vi "CAN Jaguar Get Status.vi"(8 "error in (no error)":errorcluster, 10 "Status Select":T1[](array[typedef])=[enum."Voltage"], 11 "CAN Jaguar Ref":T3={"Device Number"=0, "Control Mode"=enum."Percent VBus", "Inverted"=FALSE, "Semaphore"=refnum, "Max Vout"=12.0, "DevStatus"={"status"=FALSE, "code"=0, "source"=""}}) -> (0 "error out":errorcluster, 2 "Status":T2, 3 "CAN Jaguar Ref Out":T3={"Device Number"=0, "Control Mode"=enum."Percent VBus", "Inverted"=FALSE, "Semaphore"=refnum, "Max Vout"=12.0, "DevStatus"={"status"=FALSE, "code"=0, "source"=""}})   [LabVIEW 2009, in "CAN.lvlib"]
uses:
  CAN.lvlib
  SubVIs/CAN Jaguar Ref.ctl
  SubVIs/CAN Jaguar Control Mode.ctl
  SubVIs/CAN Jaguar Status.ctl
  SubVIs/CAN Jaguar Status Select.ctl
  SubVIs/CAN Motor Message IDs.ctl
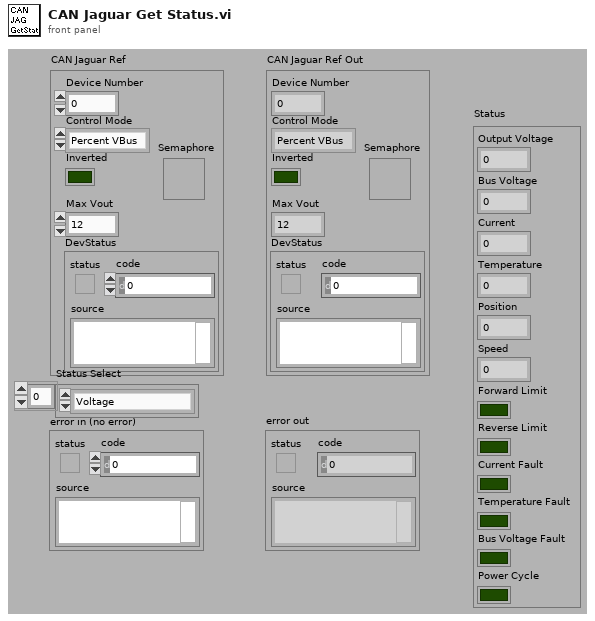
[diagram p1: front panel]
types:
  T1 = typedef "CAN.lvlib/CAN Jaguar Status Select.ctl" = enum16{"Voltage", "Current", "Temperature", "Position", "Speed", "Limit Switches", "Faults", "Power Cycle"}
  T2 = typedef "CAN.lvlib/CAN Jaguar Status.ctl" = cluster{"Output Voltage":dbl, "Bus Voltage":dbl, "Current":dbl, "Temperature":dbl, "Position":dbl, "Speed":dbl, "Forward Limit":bool, "Reverse Limit":bool, "Current Fault":bool, "Temperature Fault":bool, "Bus Voltage Fault":bool, "Power Cycle":bool}
  T3 = typedef "CAN.lvlib/CAN Jaguar Ref.ctl" = cluster{"Device Number":u8, "Control Mode":T4, "Inverted":bool, "Semaphore":T5, "Max Vout":dbl, "DevStatus":errorcluster}
  T4 = typedef "CAN.lvlib/CAN Jaguar Control Mode.ctl" = enum16{"Percent VBus", "Speed", "Position", "Current"}
  T5 = typedef "Semaphore RefNum" = refnum<k1>
  T6 = enum16{"big-endian, network order", "native, host order", "little-endian"}
  T7 = typedef "CAN Jaguar Status.ctl" = cluster{"Output Voltage":dbl, "Bus Voltage":dbl, "Current":dbl, "Temperature":dbl, "Position":dbl, "Speed":dbl, "Forward Limit":bool, "Reverse Limit":bool, "Current Fault":bool, "Temperature Fault":bool, "Bus Voltage Fault":bool, "Power Cycle":bool}
  T8 = typedef "CAN.lvlib/CAN Motor Message IDs.ctl" = u32
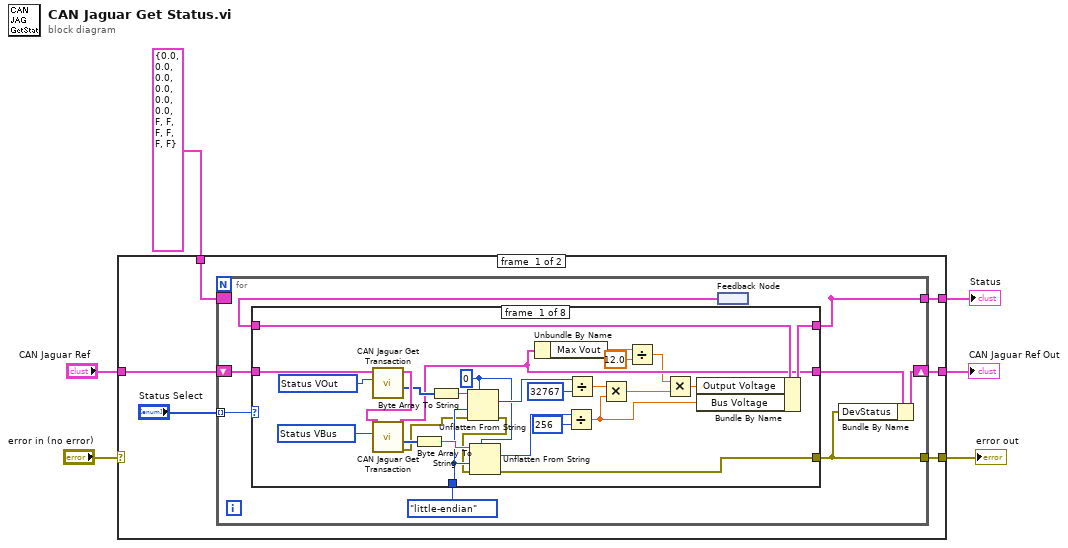
[diagram p0: block diagram]
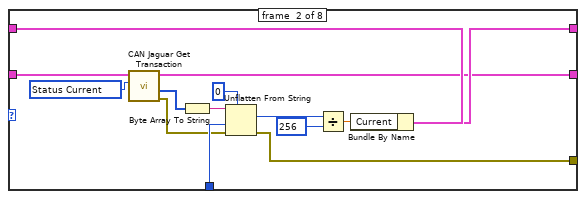
[diagram p2: hidden frame]
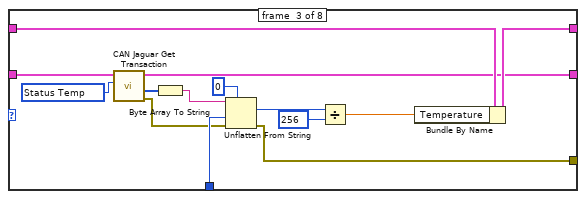
[diagram p3: hidden frame]
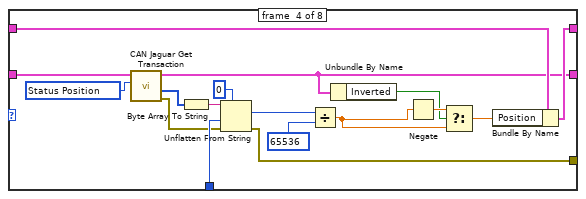
[diagram p4: hidden frame]
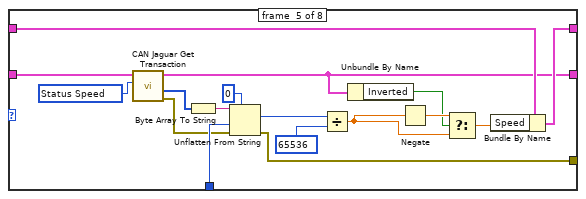
[diagram p5: hidden frame]
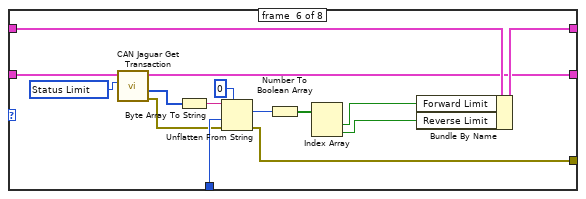
[diagram p6: hidden frame]
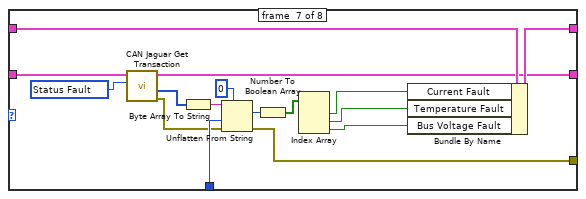
[diagram p7: hidden frame]
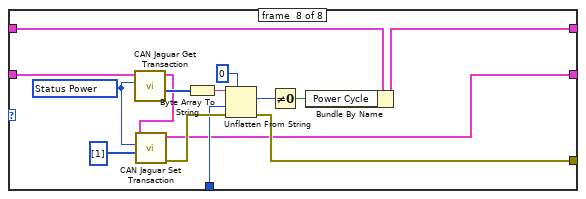
[diagram p8: hidden frame]
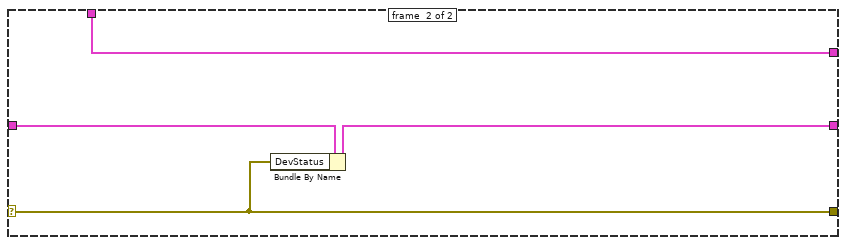
[diagram p9: hidden frame]
diagram:
  n1 = case shown="No Error" "error in (no error)" {
    selector: "error in (no error)" -> [_ w157]
    tunnel: [w7 w158] -> w6
    tunnel: "CAN Jaguar Ref" -> [w8 w159]
    tunnel: [w12 w157] -> w4
    tunnel: T2 {"Output Voltage"=0.0, "Bus Voltage"=0.0, "Current"=0.0, "Temperature"=0.0, "Position"=0.0, "Speed"=0.0, "Forward Limit"=FALSE, "Reverse Limit"=FALSE, "Current Fault"=FALSE, "Temperature Fault"=FALSE, "Bus Voltage Fault"=FALSE, "Power Cycle"=FALSE} ("Status") -> [w10 w156]
    tunnel: [w9 w156] -> w1
    frame #0 {
      n2 = for {
        tunnel: [w15] -> w12
        tunnel: "Status Select" -> [w20] mode=indexing
        border: w10 -> [_]
        tunnel: [w17] -> w9
        shift-right: [w13] -> w7
        shift-left: w8 -> [w16]
        n3 = feedback #1() -> (w19:T7)
        n4 = case shown="\"Current\"" w20 {
          tunnel: T6."little-endian" ("byte order (0:big-endian, network order)") -> [w29 w61 w75 w92 w109 w124 w140 w143]
          tunnel: [w47 w59 w73 w90 w107 w122 w138 w144] -> w15
          tunnel: w19 -> [w45 w58 w70 w89 w106 w121 w137 w155]
          tunnel: [w44 w57 w69 w88 w105 w120 w136 w154] -> w17
          tunnel: w16 -> [w34 w50 w67 w81 w98 w112 w127 w145]
          tunnel: [w25 w48 w62 w77 w94 w110 w125 w141] -> w14
          frame #0 {
            w27 = i16 0 ("Voltage")
            w35 = T8 33690624 items=["Volt Enable"=33685504, "Volt Disable"=33685568, "Volt Set"=33685632, "Volt Set Ramp"=33685696, "Speed Enable"=33686528, "Speed Disable"=33686592, "Speed Set"=33686656, "Speed P"=33686720, "Speed I"=33686784, "Speed D"=33686848, "Speed Ref"=33686912, "Position Enable"=33688576, "Position Disable"=33688640, "Position Set"=33688704, "Position P"=33688768, "Position I"=33688832, "Position D"=33688896, "Position Ref"=33688960, "Current Enable"=33689600, "Current Disable"=33689664, "Current Set"=33689728, "Current P"=33689792, "Current I"=33689856, "Current D"=33689920, "Status VOut"=33690624, "Status VBus"=33690688, "Status Current"=33690752, "Status Temp"=33690816, "Status Position"=33690880, "Status Speed"=33690944, "Status Limit"=33691008, "Status Fault"=33691072, "Status Power"=33691136, "Config Num Brushes"=33692672, "Config Encoder Lines"=33692736, "Config Pot Turns"=33692800, "Config Brake Coast"=33692864, "Config Limit Mode"=33692928, "Config Limit Fwd"=33692992, "Config Limit Rev"=33693056, "Config Max VOut"=33693120, "Config Fault Time"=33693184, "Motor Ack"=33693696] ("CAN Motor Message IDs")
            w36 = T8 33690688 items=["Volt Enable"=33685504, "Volt Disable"=33685568, "Volt Set"=33685632, "Volt Set Ramp"=33685696, "Speed Enable"=33686528, "Speed Disable"=33686592, "Speed Set"=33686656, "Speed P"=33686720, "Speed I"=33686784, "Speed D"=33686848, "Speed Ref"=33686912, "Position Enable"=33688576, "Position Disable"=33688640, "Position Set"=33688704, "Position P"=33688768, "Position I"=33688832, "Position D"=33688896, "Position Ref"=33688960, "Current Enable"=33689600, "Current Disable"=33689664, "Current Set"=33689728, "Current P"=33689792, "Current I"=33689856, "Current D"=33689920, "Status VOut"=33690624, "Status VBus"=33690688, "Status Current"=33690752, "Status Temp"=33690816, "Status Position"=33690880, "Status Speed"=33690944, "Status Limit"=33691008, "Status Fault"=33691072, "Status Power"=33691136, "Config Num Brushes"=33692672, "Config Encoder Lines"=33692736, "Config Pot Turns"=33692800, "Config Brake Coast"=33692864, "Config Limit Mode"=33692928, "Config Limit Fwd"=33692992, "Config Limit Rev"=33693056, "Config Max VOut"=33693120, "Config Fault Time"=33693184, "Motor Ack"=33693696] ("CAN Motor Message IDs")
            n5 = call "CAN Jaguar Get Transaction.vi"("Message ID"=w35, "CAN Jaguar Ref"=w34) -> ("Data"=w31:u8[], "CAN Jaguar Ref Out"=w33:T3)  [unwired: 1 in, 7 out]
            n6 = call "CAN Jaguar Get Transaction.vi"("Message ID"=w36, "CAN Jaguar Ref"=w33) -> ("error out"=w28:errorcluster, "Data"=w37:u8[], "CAN Jaguar Ref Out"=w25:T3)  [unwired: 1 in, 6 out]
            n7 = Byte Array To String(unsigned byte array=w37) -> (string=w38:string)
            n8 = Byte Array To String(unsigned byte array=w31) -> (string=w32:string)
            n9 = Unflatten From String(type=w27, binary string=w32, byte order (0:big-endian, network order)=w29, error in (no error)=w28) -> (value=w30:i16, error out=w26:errorcluster)  [unwired: 2 out]
            n10 = Unflatten From String(type=w27, binary string=w38, byte order (0:big-endian, network order)=w29, error in (no error)=w26) -> (value=w43:i16, error out=w47:errorcluster)  [unwired: 2 out]
            n11 = Unbundle By Name(w25) -> ("Max Vout"=w23:dbl)
            n12 = Divide(x=w43, y=i16 256) -> (x/y=w40:dbl)
            n13 = Divide(x=w30, y=i16 32767) -> (x/y=w39:dbl)
            n14 = Multiply(x=w39, y=w40) -> (x*y=w41:dbl)
            n15 = Divide(x=w23, y=12.0) -> (x/y=w21:dbl)
            n16 = Multiply(x=w21, y=w41) -> (x*y=w24:dbl)
            n17 = Bundle By Name(cluster=w45, "Output Voltage"=w24, "Bus Voltage"=w40) -> (w44:T7)
          }
          frame #1 {
            w49 = T8 33690752 items=["Volt Enable"=33685504, "Volt Disable"=33685568, "Volt Set"=33685632, "Volt Set Ramp"=33685696, "Speed Enable"=33686528, "Speed Disable"=33686592, "Speed Set"=33686656, "Speed P"=33686720, "Speed I"=33686784, "Speed D"=33686848, "Speed Ref"=33686912, "Position Enable"=33688576, "Position Disable"=33688640, "Position Set"=33688704, "Position P"=33688768, "Position I"=33688832, "Position D"=33688896, "Position Ref"=33688960, "Current Enable"=33689600, "Current Disable"=33689664, "Current Set"=33689728, "Current P"=33689792, "Current I"=33689856, "Current D"=33689920, "Status VOut"=33690624, "Status VBus"=33690688, "Status Current"=33690752, "Status Temp"=33690816, "Status Position"=33690880, "Status Speed"=33690944, "Status Limit"=33691008, "Status Fault"=33691072, "Status Power"=33691136, "Config Num Brushes"=33692672, "Config Encoder Lines"=33692736, "Config Pot Turns"=33692800, "Config Brake Coast"=33692864, "Config Limit Mode"=33692928, "Config Limit Fwd"=33692992, "Config Limit Rev"=33693056, "Config Max VOut"=33693120, "Config Fault Time"=33693184, "Motor Ack"=33693696] ("CAN Motor Message IDs")
            n18 = call "CAN Jaguar Get Transaction.vi"("Message ID"=w49, "CAN Jaguar Ref"=w50) -> ("error out"=w51:errorcluster, "Data"=w52:u8[], "CAN Jaguar Ref Out"=w48:T3)  [unwired: 1 in, 6 out]
            n19 = Byte Array To String(unsigned byte array=w52) -> (string=w53:string)
            n20 = Unflatten From String(type=i16 0 ("Voltage"), binary string=w53, byte order (0:big-endian, network order)=w61, error in (no error)=w51) -> (value=w56:i16, error out=w59:errorcluster)  [unwired: 2 out]
            n21 = Divide(x=w56, y=256) -> (x/y=w54:dbl)
            n22 = Bundle By Name(cluster=w58, "Current"=w54) -> (w57:T7)
          }
          frame #2 {
            w64 = T8 33690816 items=["Volt Enable"=33685504, "Volt Disable"=33685568, "Volt Set"=33685632, "Volt Set Ramp"=33685696, "Speed Enable"=33686528, "Speed Disable"=33686592, "Speed Set"=33686656, "Speed P"=33686720, "Speed I"=33686784, "Speed D"=33686848, "Speed Ref"=33686912, "Position Enable"=33688576, "Position Disable"=33688640, "Position Set"=33688704, "Position P"=33688768, "Position I"=33688832, "Position D"=33688896, "Position Ref"=33688960, "Current Enable"=33689600, "Current Disable"=33689664, "Current Set"=33689728, "Current P"=33689792, "Current I"=33689856, "Current D"=33689920, "Status VOut"=33690624, "Status VBus"=33690688, "Status Current"=33690752, "Status Temp"=33690816, "Status Position"=33690880, "Status Speed"=33690944, "Status Limit"=33691008, "Status Fault"=33691072, "Status Power"=33691136, "Config Num Brushes"=33692672, "Config Encoder Lines"=33692736, "Config Pot Turns"=33692800, "Config Brake Coast"=33692864, "Config Limit Mode"=33692928, "Config Limit Fwd"=33692992, "Config Limit Rev"=33693056, "Config Max VOut"=33693120, "Config Fault Time"=33693184, "Motor Ack"=33693696] ("CAN Motor Message IDs")
            n23 = call "CAN Jaguar Get Transaction.vi"("Message ID"=w64, "CAN Jaguar Ref"=w67) -> ("error out"=w63:errorcluster, "Data"=w66:u8[], "CAN Jaguar Ref Out"=w62:T3)  [unwired: 1 in, 6 out]
            n24 = Byte Array To String(unsigned byte array=w66) -> (string=w65:string)
            n25 = Unflatten From String(type=i16 0 ("Voltage"), binary string=w65, byte order (0:big-endian, network order)=w75, error in (no error)=w63) -> (value=w72:i16, error out=w73:errorcluster)  [unwired: 2 out]
            n26 = Divide(x=w72, y=256) -> (x/y=w68:dbl)
            n27 = Bundle By Name(cluster=w70, "Temperature"=w68) -> (w69:T7)
          }
          frame #3 {
            w84 = T8 33690880 items=["Volt Enable"=33685504, "Volt Disable"=33685568, "Volt Set"=33685632, "Volt Set Ramp"=33685696, "Speed Enable"=33686528, "Speed Disable"=33686592, "Speed Set"=33686656, "Speed P"=33686720, "Speed I"=33686784, "Speed D"=33686848, "Speed Ref"=33686912, "Position Enable"=33688576, "Position Disable"=33688640, "Position Set"=33688704, "Position P"=33688768, "Position I"=33688832, "Position D"=33688896, "Position Ref"=33688960, "Current Enable"=33689600, "Current Disable"=33689664, "Current Set"=33689728, "Current P"=33689792, "Current I"=33689856, "Current D"=33689920, "Status VOut"=33690624, "Status VBus"=33690688, "Status Current"=33690752, "Status Temp"=33690816, "Status Position"=33690880, "Status Speed"=33690944, "Status Limit"=33691008, "Status Fault"=33691072, "Status Power"=33691136, "Config Num Brushes"=33692672, "Config Encoder Lines"=33692736, "Config Pot Turns"=33692800, "Config Brake Coast"=33692864, "Config Limit Mode"=33692928, "Config Limit Fwd"=33692992, "Config Limit Rev"=33693056, "Config Max VOut"=33693120, "Config Fault Time"=33693184, "Motor Ack"=33693696] ("CAN Motor Message IDs")
            n28 = call "CAN Jaguar Get Transaction.vi"("Message ID"=w84, "CAN Jaguar Ref"=w81) -> ("error out"=w83:errorcluster, "Data"=w82:u8[], "CAN Jaguar Ref Out"=w77:T3)  [unwired: 1 in, 6 out]
            n29 = Byte Array To String(unsigned byte array=w82) -> (string=w85:string)
            n30 = Unflatten From String(type=0 ("Voltage"), binary string=w85, byte order (0:big-endian, network order)=w92, error in (no error)=w83) -> (value=w87:i32, error out=w90:errorcluster)  [unwired: 2 out]
            n31 = Divide(x=w87, y=65536 ("value")) -> (x/y=w78:dbl)
            n32 = Unbundle By Name(w77) -> ("Inverted"=w76:bool)
            n33 = Negate(x=w78) -> (-x=w79:dbl)
            n34 = Select(t=w79, s=w76, f=w78) -> (s? t:f=w80:dbl)
            n35 = Bundle By Name(cluster=w89, "Position"=w80) -> (w88:T7)
          }
          frame #4 {
            w99 = T8 33690944 items=["Volt Enable"=33685504, "Volt Disable"=33685568, "Volt Set"=33685632, "Volt Set Ramp"=33685696, "Speed Enable"=33686528, "Speed Disable"=33686592, "Speed Set"=33686656, "Speed P"=33686720, "Speed I"=33686784, "Speed D"=33686848, "Speed Ref"=33686912, "Position Enable"=33688576, "Position Disable"=33688640, "Position Set"=33688704, "Position P"=33688768, "Position I"=33688832, "Position D"=33688896, "Position Ref"=33688960, "Current Enable"=33689600, "Current Disable"=33689664, "Current Set"=33689728, "Current P"=33689792, "Current I"=33689856, "Current D"=33689920, "Status VOut"=33690624, "Status VBus"=33690688, "Status Current"=33690752, "Status Temp"=33690816, "Status Position"=33690880, "Status Speed"=33690944, "Status Limit"=33691008, "Status Fault"=33691072, "Status Power"=33691136, "Config Num Brushes"=33692672, "Config Encoder Lines"=33692736, "Config Pot Turns"=33692800, "Config Brake Coast"=33692864, "Config Limit Mode"=33692928, "Config Limit Fwd"=33692992, "Config Limit Rev"=33693056, "Config Max VOut"=33693120, "Config Fault Time"=33693184, "Motor Ack"=33693696] ("CAN Motor Message IDs")
            n36 = call "CAN Jaguar Get Transaction.vi"("Message ID"=w99, "CAN Jaguar Ref"=w98) -> ("error out"=w100:errorcluster, "Data"=w101:u8[], "CAN Jaguar Ref Out"=w94:T3)  [unwired: 1 in, 6 out]
            n37 = Byte Array To String(unsigned byte array=w101) -> (string=w102:string)
            n38 = Unflatten From String(type=0 ("Voltage"), binary string=w102, byte order (0:big-endian, network order)=w109, error in (no error)=w100) -> (value=w103:i32, error out=w107:errorcluster)  [unwired: 2 out]
            n39 = Divide(x=w103, y=65536 ("value")) -> (x/y=w95:dbl)
            n40 = Unbundle By Name(w94) -> ("Inverted"=w93:bool)
            n41 = Negate(x=w95) -> (-x=w96:dbl)
            n42 = Select(t=w96, s=w93, f=w95) -> (s? t:f=w97:dbl)
            n43 = Bundle By Name(cluster=w106, "Speed"=w97) -> (w105:T7)
          }
          frame #5 {
            w111 = T8 33691008 items=["Volt Enable"=33685504, "Volt Disable"=33685568, "Volt Set"=33685632, "Volt Set Ramp"=33685696, "Speed Enable"=33686528, "Speed Disable"=33686592, "Speed Set"=33686656, "Speed P"=33686720, "Speed I"=33686784, "Speed D"=33686848, "Speed Ref"=33686912, "Position Enable"=33688576, "Position Disable"=33688640, "Position Set"=33688704, "Position P"=33688768, "Position I"=33688832, "Position D"=33688896, "Position Ref"=33688960, "Current Enable"=33689600, "Current Disable"=33689664, "Current Set"=33689728, "Current P"=33689792, "Current I"=33689856, "Current D"=33689920, "Status VOut"=33690624, "Status VBus"=33690688, "Status Current"=33690752, "Status Temp"=33690816, "Status Position"=33690880, "Status Speed"=33690944, "Status Limit"=33691008, "Status Fault"=33691072, "Status Power"=33691136, "Config Num Brushes"=33692672, "Config Encoder Lines"=33692736, "Config Pot Turns"=33692800, "Config Brake Coast"=33692864, "Config Limit Mode"=33692928, "Config Limit Fwd"=33692992, "Config Limit Rev"=33693056, "Config Max VOut"=33693120, "Config Fault Time"=33693184, "Motor Ack"=33693696] ("CAN Motor Message IDs")
            n44 = call "CAN Jaguar Get Transaction.vi"("Message ID"=w111, "CAN Jaguar Ref"=w112) -> ("error out"=w114:errorcluster, "Data"=w113:u8[], "CAN Jaguar Ref Out"=w110:T3)  [unwired: 1 in, 6 out]
            n45 = Byte Array To String(unsigned byte array=w113) -> (string=w115:string)
            n46 = Unflatten From String(type=u8 0 ("Voltage"), binary string=w115, byte order (0:big-endian, network order)=w124, error in (no error)=w114) -> (value=w119:u8, error out=w122:errorcluster)  [unwired: 2 out]
            n47 = Number To Boolean Array(number=w119) -> (Boolean array=w118:bool[])
            n48 = Index Array(array=w118) -> (element #1=w117:bool, element #2=w116:bool)  [unwired: 2 in]
            n49 = Bundle By Name(cluster=w121, "Forward Limit"=w117, "Reverse Limit"=w116) -> (w120:T7)
          }
          frame #6 {
            w126 = T8 33691072 items=["Volt Enable"=33685504, "Volt Disable"=33685568, "Volt Set"=33685632, "Volt Set Ramp"=33685696, "Speed Enable"=33686528, "Speed Disable"=33686592, "Speed Set"=33686656, "Speed P"=33686720, "Speed I"=33686784, "Speed D"=33686848, "Speed Ref"=33686912, "Position Enable"=33688576, "Position Disable"=33688640, "Position Set"=33688704, "Position P"=33688768, "Position I"=33688832, "Position D"=33688896, "Position Ref"=33688960, "Current Enable"=33689600, "Current Disable"=33689664, "Current Set"=33689728, "Current P"=33689792, "Current I"=33689856, "Current D"=33689920, "Status VOut"=33690624, "Status VBus"=33690688, "Status Current"=33690752, "Status Temp"=33690816, "Status Position"=33690880, "Status Speed"=33690944, "Status Limit"=33691008, "Status Fault"=33691072, "Status Power"=33691136, "Config Num Brushes"=33692672, "Config Encoder Lines"=33692736, "Config Pot Turns"=33692800, "Config Brake Coast"=33692864, "Config Limit Mode"=33692928, "Config Limit Fwd"=33692992, "Config Limit Rev"=33693056, "Config Max VOut"=33693120, "Config Fault Time"=33693184, "Motor Ack"=33693696] ("CAN Motor Message IDs")
            n50 = call "CAN Jaguar Get Transaction.vi"("Message ID"=w126, "CAN Jaguar Ref"=w127) -> ("error out"=w129:errorcluster, "Data"=w128:u8[], "CAN Jaguar Ref Out"=w125:T3)  [unwired: 1 in, 6 out]
            n51 = Byte Array To String(unsigned byte array=w128) -> (string=w130:string)
            n52 = Unflatten From String(type=u16 0 ("Voltage"), binary string=w130, byte order (0:big-endian, network order)=w140, error in (no error)=w129) -> (value=w135:u16, error out=w138:errorcluster)  [unwired: 2 out]
            n53 = Number To Boolean Array(number=w135) -> (Boolean array=w134:bool[])
            n54 = Index Array(array=w134) -> (element #1=w133:bool, element #2=w132:bool, element #3=w131:bool)  [unwired: 3 in]
            n55 = Bundle By Name(cluster=w137, "Current Fault"=w133, "Temperature Fault"=w132, "Bus Voltage Fault"=w131) -> (w136:T7)
          }
          frame #7 {
            w150 = T8 33691136 items=["Volt Enable"=33685504, "Volt Disable"=33685568, "Volt Set"=33685632, "Volt Set Ramp"=33685696, "Speed Enable"=33686528, "Speed Disable"=33686592, "Speed Set"=33686656, "Speed P"=33686720, "Speed I"=33686784, "Speed D"=33686848, "Speed Ref"=33686912, "Position Enable"=33688576, "Position Disable"=33688640, "Position Set"=33688704, "Position P"=33688768, "Position I"=33688832, "Position D"=33688896, "Position Ref"=33688960, "Current Enable"=33689600, "Current Disable"=33689664, "Current Set"=33689728, "Current P"=33689792, "Current I"=33689856, "Current D"=33689920, "Status VOut"=33690624, "Status VBus"=33690688, "Status Current"=33690752, "Status Temp"=33690816, "Status Position"=33690880, "Status Speed"=33690944, "Status Limit"=33691008, "Status Fault"=33691072, "Status Power"=33691136, "Config Num Brushes"=33692672, "Config Encoder Lines"=33692736, "Config Pot Turns"=33692800, "Config Brake Coast"=33692864, "Config Limit Mode"=33692928, "Config Limit Fwd"=33692992, "Config Limit Rev"=33693056, "Config Max VOut"=33693120, "Config Fault Time"=33693184, "Motor Ack"=33693696] ("CAN Motor Message IDs")
            n56 = call "CAN Jaguar Get Transaction.vi"("Message ID"=w150, "CAN Jaguar Ref"=w145) -> ("Data"=w151:u8[], "CAN Jaguar Ref Out"=w142:T3)  [unwired: 1 in, 7 out]
            n57 = call "CAN Jaguar Set Transaction.vi"("Data"=u8[] [1] ("data"), "Message ID"=w150, "CAN Jaguar Ref"=w142) -> ("error out"=w152:errorcluster, "CAN Jaguar Ref Out"=w141:T3)  [unwired: 1 in, 6 out]
            n58 = Byte Array To String(unsigned byte array=w151) -> (string=w147:string)
            n59 = Unflatten From String(type=u8 0 ("Voltage"), binary string=w147, byte order (0:big-endian, network order)=w143, error in (no error)=w152) -> (value=w146:u8, error out=w144:errorcluster)  [unwired: 2 out]
            n60 = Not Equal To 0?(x=w146) -> (x != 0?=w153:bool)
            n61 = Bundle By Name(cluster=w155, "Power Cycle"=w153) -> (w154:T7)
          }
        }
        n62 = Bundle By Name(cluster=w14, "DevStatus"=w15) -> (w13:T3)
      }
    }
    frame #1 {
      n63 = Bundle By Name(cluster=w159, "DevStatus"=w157) -> (w158:T3)
    }
  }
  "CAN Jaguar Ref Out" <- w6
  "error out" <- w4
  "Status" <- w1
